vi "8164B SendString.vi"(8 "error in":errorcluster, 10 "CMD":string, 11 "KeySight 8164B control in":T1) -> (0 "error out":errorcluster, 3 "KeySight 8164B control out":T1)   [LabVIEW 2018, in "KeySight 8164B LAN InstrLib.lvlib"]
uses:
  KeySight 8164B LAN InstrLib.lvlib
  typedefs/KeySight 8164B control.ctl
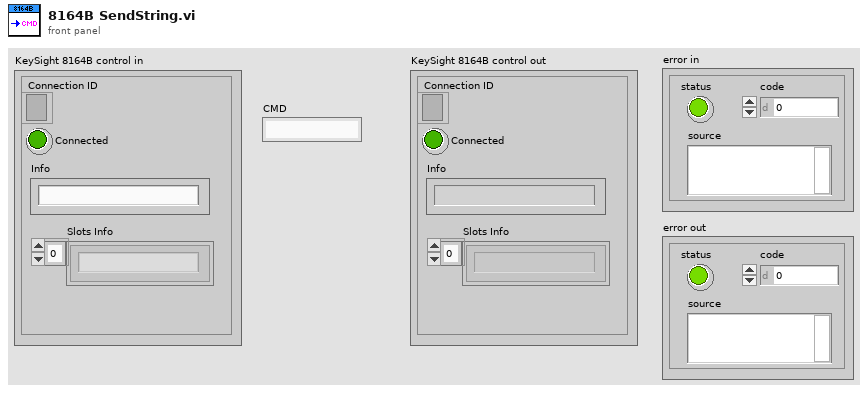
[diagram p1: front panel]
types:
  T1 = typedef "KeySight 8164B LAN InstrLib.lvlib/KeySight 8164B control.ctl" = cluster{"Connection ID":refnum<k5>, "Connected":bool, "Info":string, "Slots Info":string[]}
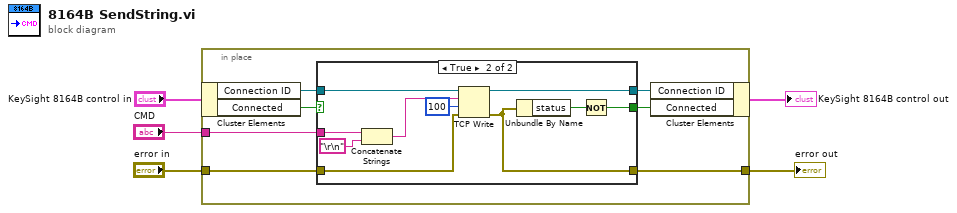
[diagram p0: block diagram]
diagram:
  n1 = in-place {
    in-place-border: "CMD" -> [w10]
    in-place-border: "error in" -> [w9]
    in-place-border: [w8] -> w1
    n2 = in-place-cluster #1("KeySight 8164B control in") -> ("Connection ID"=w12:refnum<k5>, "Connected"=w6:bool)
    n3 = case shown="True" w6 {
      selector: w6 -> [w13 _]
      tunnel: w12 -> [w14 w25]
      tunnel: [w14 w24] -> w11
      tunnel: w10 -> [_ w23]
      tunnel: w9 -> [w15 w22]
      tunnel: [w15 w20] -> w8
      tunnel: [w13 w19] -> w7
      frame False {
      }
      frame True {
        n4 = Concatenate Strings(w23, "\r\n") -> (w17:string)
        n5 = TCP Write(connection ID=w25, data in=w17, error in (no error)=w22, 9:100 ("timeout ms (25000)")) -> (connection ID out=w24:refnum<k5>, error out=w20:errorcluster)  [unwired: 1 out]
        n6 = Unbundle By Name(w20) -> ("status"=w21:bool)
        n7 = Not(x=w21) -> (.not. x?=w19:bool)
      }
    }
    n8 = in-place-cluster #1("Connection ID"=w11, "Connected"=w7) -> (→"KeySight 8164B control out":T1)
  }
  "error out" <- w1
